vi "Get Tweets New.vi"(8 "error in":errorcluster, 9 "Tweets to Read (10)":i32=10 min=0 max=200 step=1, 10 "Screen Name (Empty)":string, 11 "Twitter Handle In":T2={"OAuth Credentials"={"Signature Method"=enum."HMAC-SHA1", "Version"="1.0", "Client"={"Token"="", "Secret"=""}, "Access"={"Token"="", "Secret"=""}}, "since ID"="", "max ID"="", "Screen Name"=""}) -> (0 "error out":errorcluster, 1 "Actual Num of Tweets Read":i32, 2 "New Tweets Read":T1[](array[typedef]), 3 "Twitter Handle Out":T2={"OAuth Credentials"={"Signature Method"=enum."HMAC-SHA1", "Version"="1.0", "Client"={"Token"="", "Secret"=""}, "Access"={"Token"="", "Secret"=""}}, "since ID"="", "max ID"="", "Screen Name"=""}, 5 "Time Stamp of Newest Tweet":timestamp)   [LabVIEW 2011, in "i3-twitter.lvlib"]
doc: "Get new tweets for the screen name. If no screen name is provided, tweets for the authenticating user are returned."
uses:
  i3-twitter.lvlib
  Controls/Twitter Handle.ctl
  i3-oauth/Controls/OAuth Handle.ctl
  i3-oauth/Controls/Signature Method.ctl
  i3-oauth/Controls/Credentials.ctl
  Controls/Tweet.ctl
  i3-oauth/Controls/HTTP Method.ctl
  i3-json/JSON Parsing/Get Array Value at Index Files/Get Array Value at Index - Object.vi
  i3-json/JSON Parsing/Get Object Parameter Files/Get Object Parameter - String.vi
  i3-json/JSON Parsing/Get Object Parameter Files/Get Object Parameter - Object.vi
  i3-oauth/i3-oauth.lvlib
  <vilib>/httpClient/LabVIEWHTTPClient.lvlib
  i3-json/i3-json.lvlib
panel:
  out "headers":string
  out "body":string
  out "Full URL":string
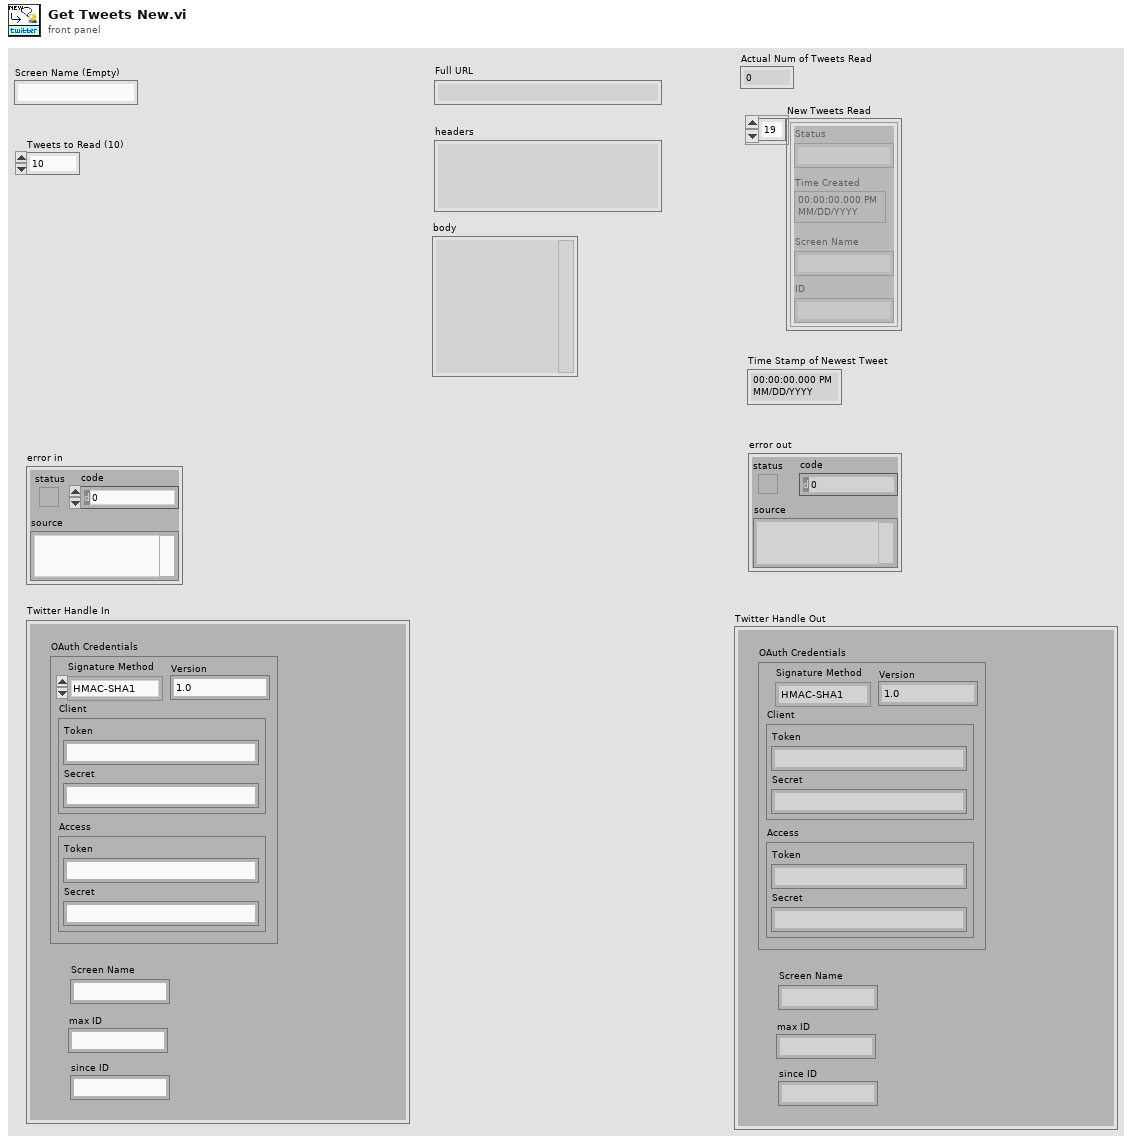
[diagram p1: front panel]
types:
  T1 = typedef "i3-twitter.lvlib/Tweet.ctl" = cluster{"Status":string, "Time Created":timestamp, "Screen Name":string, "ID":string}
  T2 = typedef "i3-twitter.lvlib/Twitter Handle.ctl" = cluster{"OAuth Credentials":T3, "since ID":string, "max ID":string, "Screen Name":string}
  T3 = typedef "i3-oauth.lvlib/OAuth Handle.ctl" = cluster{"Signature Method":T4, "Version":string, "Client":T5, "Access":T5}
  T4 = typedef "i3-oauth.lvlib/Signature Method.ctl" = enum16{"HMAC-MD5", "HMAC-SHA1", "HMAC-SHA224", "HMAC-SHA256", "HMAC-SHA384", "HMAC-SHA512"}
  T5 = typedef "i3-oauth.lvlib/Credentials.ctl" = cluster{"Token":string, "Secret":string}
  T6 = typedef "i3-oauth.lvlib/HTTP Method.ctl" = enum16{"GET", "POST", "PUT", "DELETE"}
  T7 = typedef "i3-oauth.lvlib/Name-Value Pair.ctl" = cluster{"Name":string, "Value":string}
  T8 = typedef "LabVIEWHTTPClient.lvlib/ClientHandle.ctl" = refnum<k1>
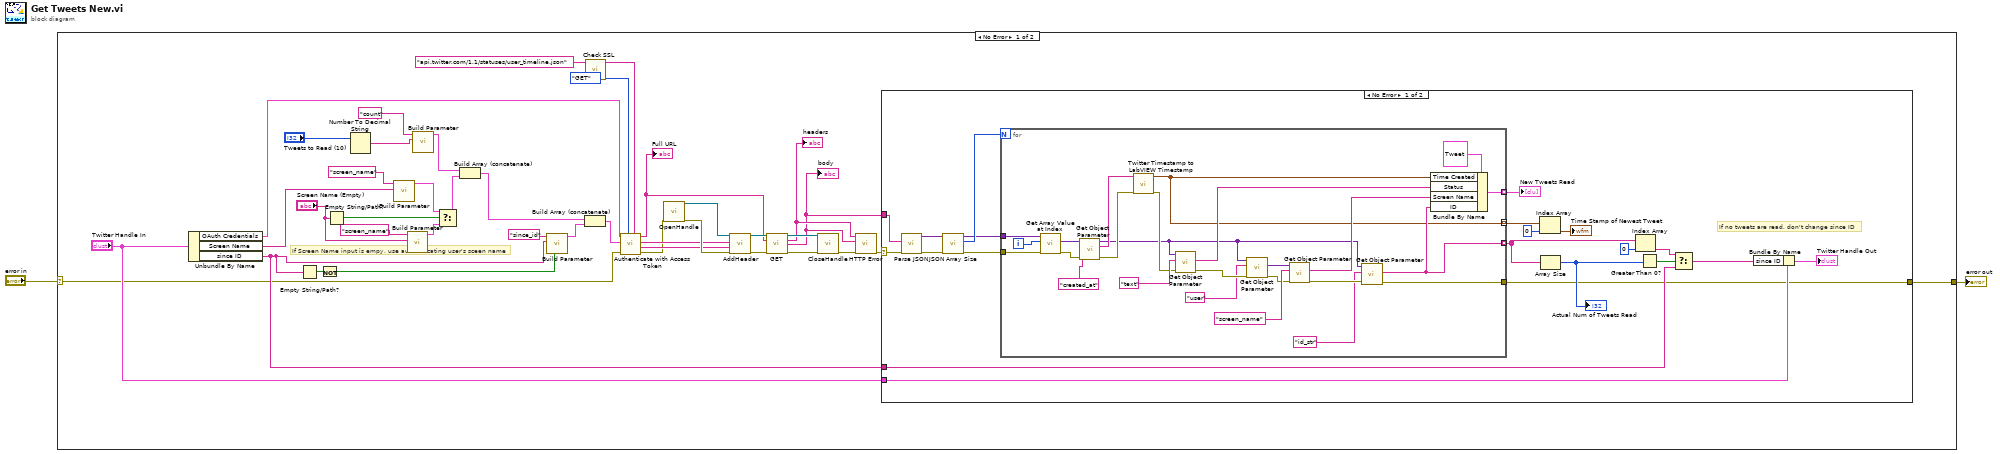
[diagram p0: block diagram]
diagram:
  n1 = case shown="No Error" "error in" {
    selector: "error in" -> [w7 w90]
    tunnel: [w11 w90] -> w2
    frame No Error {
      # "If Screen Name input is empy, use authenticating user's sceen name"
      n2 = Unbundle By Name("Twitter Handle In") -> ("OAuth Credentials"=w3:T3, "Screen Name"=w8:string, "since ID"=w9:string)
      n3 = Empty String/Path?(string/path=w9) -> (empty?=w25:bool)
      n4 = Not(x=w25) -> (.not. x?=w22:bool)
      n5 = Empty String/Path?(string/path="Screen Name (Empty)") -> (empty?=w19:bool)
      n6 = Number To Decimal String(number="Tweets to Read (10)") -> (decimal integer string=w31:string)  [unwired: 1 in]
      n7 = call "Build Parameter.vi"("Value"=w8, "Key"="screen_name") -> ("Parameter Array"=w17:T7[])  [unwired: 9 in]
      n8 = call "Build Parameter.vi"("Value"="Screen Name (Empty)", "Key"="screen_name") -> ("Parameter Array"=w16:T7[])  [unwired: 9 in]
      n9 = call "Build Parameter.vi"("Value"=w31, "Key"="count") -> ("Parameter Array"=w29:T7[])  [unwired: 9 in]
      n10 = Select(t=w17, s=w19, f=w16) -> (s? t:f=w18:T7[])
      n11 = Build Array (concatenate)(w29, w18) -> (w28:T7[])
      n12 = call "Build Parameter.vi"("Return Parameter? (T)"=w22, "Value"=w9, "Key"="since_id") -> ("Parameter Array"=w24:T7[])  [unwired: 8 in]
      n13 = Build Array (concatenate)(w28, w24) -> (w27:T7[])
      n14 = call "Check SSL.vi"("Input URL"="api.twitter.com/1.1/statuses/user_timeline.json" ("Base URL")) -> ("Output URL"=w4:string)  [unwired: 8 in]
      n15 = call "Authenticate with Access Token.vi"("Base URL"=w4, "HTTP Method"=HTTP_Method."GET", "error in (no error)"=w7, "URL Parameters"=w27, "OAuth Handle"=w3) -> ("error out"=w26:errorcluster, "Header Value"=w35:string, "Header Parameter"=w36:string, "Full URL"=w34:string)  [unwired: 2 in, 1 out]
      "Full URL" <- w34
      n16 = call <vilib>:"OpenHandle.vi"("error in (no error)"=w26) -> ("client handle out"=w42:T8, "error out"=w41:errorcluster)  [unwired: 13 in]
      n17 = call <vilib>:"AddHeader.vi"("client handle"=w42, "header"=w36, "value"=w35, "error in (no error)"=w41) -> ("client handle out"=w40:T8, "error out"=w39:errorcluster)  [unwired: 10 in]
      n18 = call <vilib>:"GET.vi"("client handle"=w40, "url"=w34, "error in (no error)"=w39) -> ("client handle out"=w38:T8, "headers"=w15:string, "body"=w10:string, "error out"=w37:errorcluster)  [unwired: 9 in]
      "body" <- w10
      "headers" <- w15
      n19 = call <vilib>:"CloseHandle.vi"("client handle"=w38, "error in (no error)"=w37) -> ("error out"=w14:errorcluster)  [unwired: 13 in]
      n20 = call "HTTP Error.vi"("error in (no error)"=w14, "Body"=w10, "Header"=w15) -> ("error out"=w12:errorcluster)  [unwired: 6 in, 2 out]
      n21 = case shown="No Error" w12 {
        selector: w12 -> [w49 w89]
        tunnel: w9 -> [w52 _]
        tunnel: "Twitter Handle In" -> [w51 _]
        tunnel: [w48 w89] -> w11
        tunnel: w10 -> [w47 _]
        frame No Error {
          # "If no tweets are read, don't change since ID"
          n22 = call "Parse JSON.vi"("error in (no error)"=w49, "JSON String"=w47) -> ("error out"=w60:errorcluster, "JSON Tree"=w62:variant)  [unwired: 6 in, 2 out]
          n23 = call "JSON Array Size.vi"("error in (no error)"=w60, "JSON Tree In (JSON Array)"=w62) -> ("error out"=w59:errorcluster, "Array Size"=w63:i32, "JSON Tree Passthrough (JSON Array)"=w53:variant)  [unwired: 7 in]
          n24 = for {
            N: w63 -> [_]
            tunnel: [w78] -> w61 mode=indexing
            tunnel: w59 -> [w73]
            tunnel: [w80] -> w58 mode=indexing
            tunnel: [w79] -> w48
            tunnel: w53 -> [w72]
            tunnel: [w71] -> w46 mode=indexing
            i -> [w83]
            n25 = call-poly "Get Array Value at Index.vi"("error in (no error)"=w73, "Index"=w83, "JSON Tree In (JSON Array)"=w72) -> ("error out"=w82:errorcluster, "JSON Object"=w70:variant)  [unwired: 5 in, 2 out]
            n26 = call-poly "Get Object Parameter.vi"("error in (no error)"=w82, "Parameter Name"="created_at", "JSON Tree In (JSON Object)"=w70) -> ("error out"=w66:errorcluster, "String Value"=w65:string, "JSON Tree Out Passthrough"=w64:variant)  [unwired: 5 in, 1 out]
            n27 = call "Twitter Timestamp to LabVIEW Timestamp.vi"("error in"=w66, "Twitter Time Stamp"=w65) -> ("error out"=w76:errorcluster, "LabVIEW Time Stamp"=w71:timestamp)  [unwired: 6 in]
            n28 = call-poly "Get Object Parameter.vi"("error in (no error)"=w76, "Parameter Name"="text", "JSON Tree In (JSON Object)"=w64) -> ("error out"=w77:errorcluster, "String Value"=w74:string)  [unwired: 5 in, 2 out]
            n29 = call-poly "Get Object Parameter.vi"("error in (no error)"=w77, "Parameter Name"="user", "JSON Tree In (JSON Object)"=w64) -> ("error out"=w81:errorcluster, "JSON Object"=w69:variant)  [unwired: 5 in, 2 out]
            n30 = call-poly "Get Object Parameter.vi"("error in (no error)"=w81, "Parameter Name"="screen_name", "JSON Tree In (JSON Object)"=w69) -> ("error out"=w75:errorcluster, "String Value"=w86:string)  [unwired: 5 in, 2 out]
            n31 = call-poly "Get Object Parameter.vi"("error in (no error)"=w75, "Parameter Name"="id_str", "JSON Tree In (JSON Object)"=w64) -> ("error out"=w79:errorcluster, "String Value"=w78:string)  [unwired: 5 in, 2 out]
            n32 = Bundle By Name(cluster=T1 {"Status"="", "Time Created"=timestamp(0 s since 1904-01-01), "Screen Name"="", "ID"=""}, "Time Created"=w71, "Status"=w74, "Screen Name"=w86, "ID"=w78) -> (w80:T1)
          }
          "New Tweets Read" <- w58
          n33 = Index Array(array=w46, index=0) -> (element=→"Time Stamp of Newest Tweet":timestamp)
          n34 = Array Size(array=w61) -> (size(s)=w56:i32)
          "Actual Num of Tweets Read" <- w56
          n35 = Index Array(array=w61, index=0) -> (element=w55:string)
          n36 = Greater Than 0?(x=w56) -> (x > 0?=w57:bool)
          n37 = Select(t=w55, s=w57, f=w52) -> (s? t:f=w54:string)
          n38 = Bundle By Name(cluster=w51, "since ID"=w54) -> (→"Twitter Handle Out":T2)
        }
        frame Error {
        }
      }
    }
    frame Error {
    }
  }
  "error out" <- w2
